vi "Measurement.IVCurve.ReftoDVR.vi"(10 "Ref":u32 format="%08x") -> (2 "Ref":T1)   [LabVIEW 2017, in "Measurement.IVCurve.lvclass"]
doc: "JKI State Machine Objects (SMO) 1.0.0.5\nJKI - JKI\nCopyright (c) 2016, JKI"
uses:
  Measurement.IVCurve.lvclass
  Typedefs/PrivateData--Ref.ctl
  Typedefs/PrivateData--Cluster.ctl
  Typedefs/Configuration--Cluster.ctl
  Measurement/Typedefs/Measurement.Type--Enum.ctl
  Typedefs/Configuration.Hardware--Cluster.ctl
  Measurement/Typedefs/Configuration.SMU--Cluster.ctl
  SMU/Typedefs/Configuration--Cluster.ctl
  Typedefs/Configuration.Measurement--Cluster.ctl
  Typedefs/Dependencies--Cluster.ctl
  SMU/SMU.lvclass
  LIA/LIA.lvclass
  OPM/OPM.lvclass
  OPA/OPA.lvclass
  Measurement/Measurement.lvclass
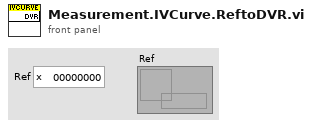
[diagram p1: front panel]
types:
  T1 = typedef "Measurement.IVCurve.lvclass/PrivateData--Ref.ctl" = refnum<data-value>
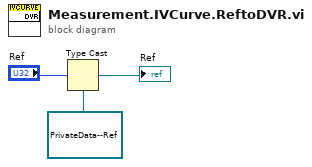
[diagram p0: block diagram]
diagram:
  n1 = Type Cast(type=T1 refnum ("Ref"), x="Ref") -> (*(type *) &x=→"Ref":T1)
